vi "toStop2.vi"(0 "Left":i16, 5 "Distance to street":dbl, 7 "Booleanos e Contadores Iniciais IN":T2={"Correct"=FALSE, "Enable State change"=TRUE, "First End"=FALSE, "Intersections crossed"=0.0, "Intersections crossed total"=0.0, "Bonecos"=0.0, "Inter correct"=FALSE} caption="Booleanos e Contadores", 11 "Right":i16) -> (3 "Boolean":bool, 8 "Booleanos e Contadores Iniciais OUT":T2={"Correct"=FALSE, "Enable State change"=TRUE, "First End"=FALSE, "Intersections crossed"=0.0, "Intersections crossed total"=0.0, "Bonecos"=0.0, "Inter correct"=FALSE} caption="Booleanos e Contadores", 12 "Enable 2":bool, 15 "CS OUT":T1(ring))   [LabVIEW 2016]
uses:
  booleanos.ctl
panel:
  # "Permite que ocorra troca \nde estados se True e interrompe-as \nse False."
  # "Booleano que retorna F quando chega em Delivery.\nGarantindo que não contará\nmais intersections"
  # "Salva o total de interseções \ncruzadas"
  # "Contador de quantas \ninterseções foram cruzadas.\nSoma ao acertar"
  # "Permite que ocorra troca \nde estados se True e interrompe-as \nse False."
  # "Booleano que retorna F quando chega em Delivery.\nGarantindo que não contará\nmais intersections"
  # "Salva o total de interseções \ncruzadas"
  # "Contador de quantas \ninterseções foram cruzadas.\nSoma ao acertar"
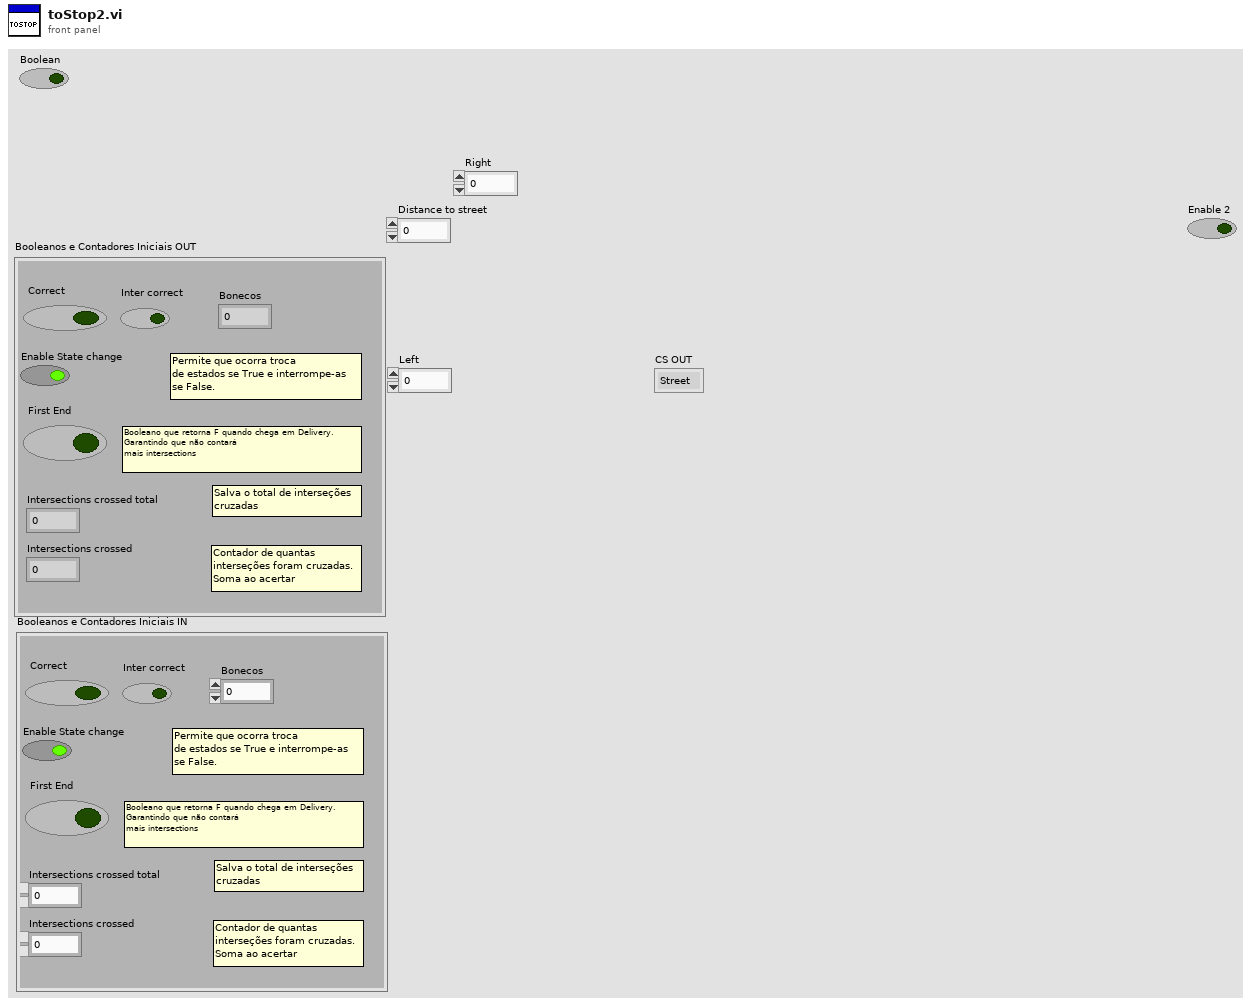
[diagram p1: front panel]
types:
  T1 = enum16{"Street", "Intersection", "End", "Stop", "Square", "Delivery", "Empty"}
  T2 = typedef "booleanos.ctl" = cluster{"Correct":bool, "Enable State change":bool, "First End":bool, "Intersections crossed":dbl, "Intersections crossed total":dbl, "Bonecos":dbl, "Inter correct":bool}
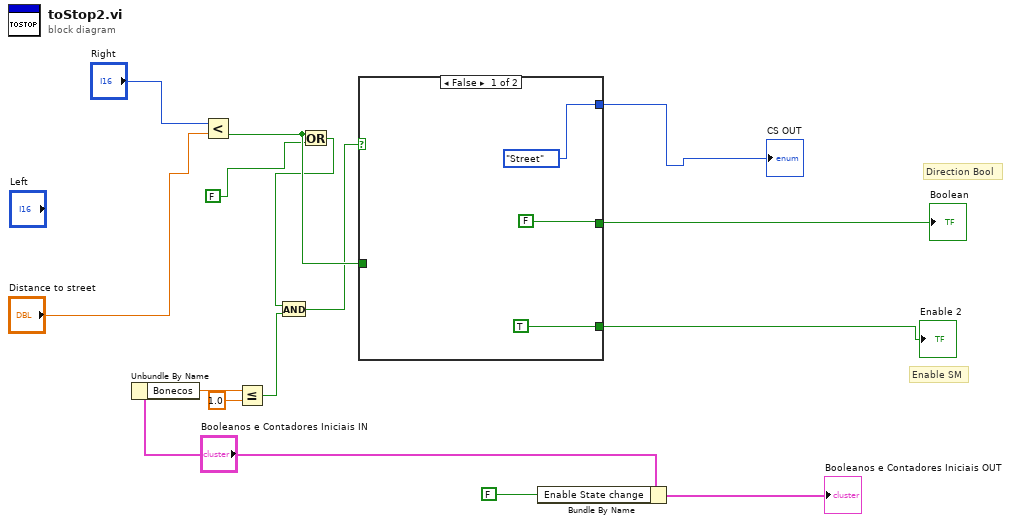
[diagram p0: block diagram]
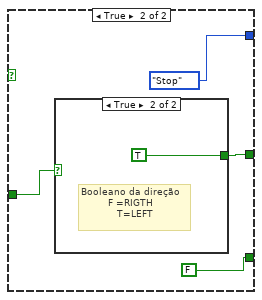
[diagram p2: hidden frame]
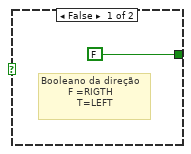
[diagram p3: hidden frame]
diagram:
  # "Enable SM"
  # "Direction Bool"
  n1 = Unbundle By Name("Booleanos e Contadores Iniciais IN") -> ("Bonecos"=w6:dbl)
  n2 = Less?(x="Right", y="Distance to street") -> (x < y?=w13:bool)
  n3 = Less Or Equal?(x=w6, y=1.0) -> (x <= y?=w4:bool)
  n4 = Or(x=w13, y=FALSE) -> (x .or. y?=w3:bool)
  n5 = And(x=w3, y=w4) -> (x .and. y?=w2:bool)
  n6 = case shown="False" w2 {
    tunnel: [T1."Street" ("CS 2") T1."Stop" ("CS 2")] -> w14
    tunnel: w13 -> [_ w22]
    tunnel: [FALSE w21] -> w12
    tunnel: [TRUE FALSE] -> w8
    frame False {
    }
    frame True {
      n7 = case shown="True" w22 {
        tunnel: [FALSE TRUE] -> w21
        frame False {
          # "Booleano da direção\n         F =RIGTH\n            T=LEFT"
        }
        frame True {
          # "Booleano da direção\n         F =RIGTH\n            T=LEFT"
        }
      }
    }
  }
  "Boolean" <- w12
  "Enable 2" <- w8
  "CS OUT" <- w14
  n8 = Bundle By Name(cluster="Booleanos e Contadores Iniciais IN", "Enable State change"=FALSE) -> (→"Booleanos e Contadores Iniciais OUT":T2)
